vi "Virtual_Blink.vi"() -> ()   [LabVIEW 2020]
uses:
  <vilib>/Instr/_visa.llb/VISA Configure Serial Port (Instr).vi
panel:
  out "x = y?":bool
  out "read buffer 2":string
  out "read buffer":string
  in  "Start":bool
  in  "Stop":bool
  in  "Serial port configuration":T1
  in  "Port":refnum<visa-resource-name>
  out "Output LED":bool
  # "Project name:  Virtual_Blink.vi \nDescription:     Blink LED emulation using Intel Galileo board\nVersion:           02.00\nRevision:          00\nLast modified : 12/31/2020"
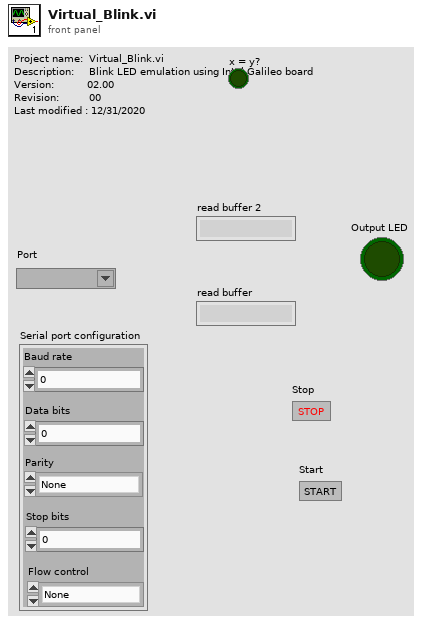
[diagram p1: front panel]
types:
  T1 = cluster{"Baud rate":u32, "Data bits":u16, "Parity":enum16{"None", "Odd", "Even", "Mark", "Space"}, "Stop bits":u16, "Flow control":enum32{"None", "XON/XOFF", "RTS/CTS", "DTR/DSR"}}
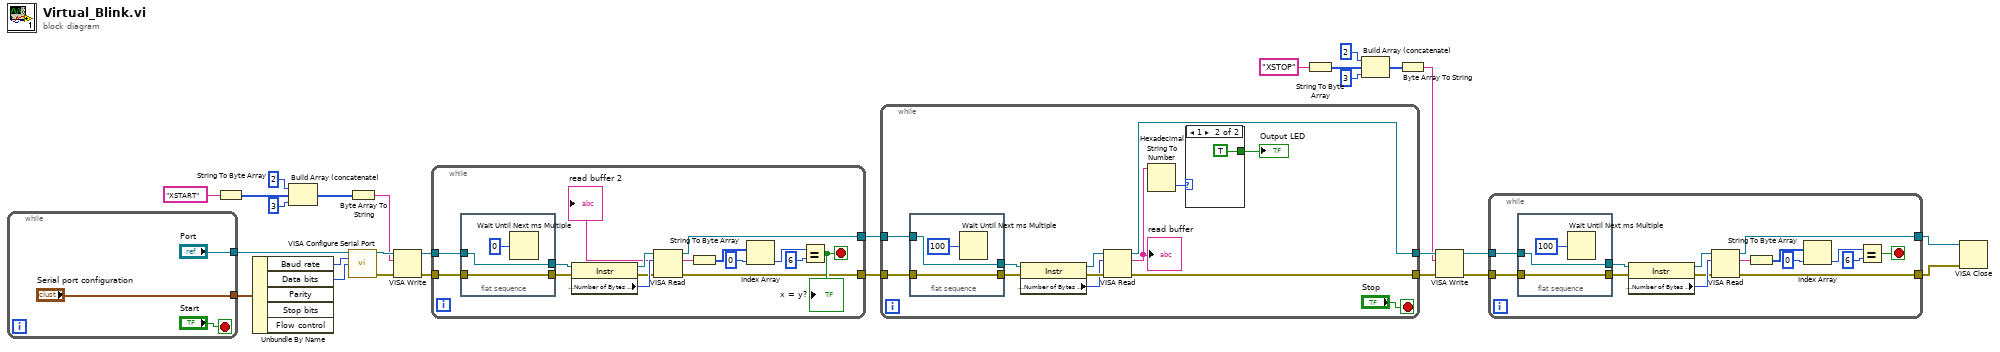
[diagram p0: block diagram]
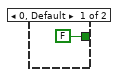
[diagram p2: hidden frame]
diagram:
  n1 = while {
    tunnel: ["Port"] -> w28
    tunnel: ["Serial port configuration"] -> w27
    stop <- "Start" stop-if-true
  }
  n2 = String To Byte Array(string="XSTART") -> (unsigned byte array=w20:u8[])
  n3 = Unbundle By Name(w27) -> ("Baud rate"=w26:u32, "Data bits"=w25:u16)  [unwired: 3 out]
  n4 = Build Array (concatenate)(u8 2, w20, u8 3) -> (w18:u8[])
  n5 = Byte Array To String(unsigned byte array=w18) -> (string=w17:string)
  n6 = call-poly "VISA Configure Serial Port"("VISA resource name"=w28, "baud rate (9600)"=w26, "data bits (8)"=w25) -> ("VISA resource name out"=w24:refnum<visa-resource-name>, "error out"=w23:errorcluster)  [unwired: 11 in]
  n7 = VISA Write(VISA resource name=w24, write buffer=w17, error in (no error)=w23) -> (VISA resource name out=w8:refnum<visa-resource-name>, error out=w7:errorcluster)  [unwired: 1 out]
  n8 = while {
    tunnel: w8 -> [w41]
    tunnel: w7 -> [w40]
    tunnel: [w33] -> w6
    tunnel: [w32] -> w5
    stop <- w34 stop-if-true
    n9 = flat-sequence {
      tunnel: w41 -> [w49]
      tunnel: w40 -> [w48]
      tunnel: [w49] -> w45
      tunnel: [w48] -> w46
      frame #0 {
        n10 = Wait Until Next ms Multiple(millisecond multiple=u32 0) -> ()  [unwired: 1 out]
      }
    }
    n11 = property class="Instr"(reference=w45, error in=w46) -> (reference out=w42:refnum<visa-resource-name>, error out=w43:errorcluster, "Serial Settings:Number of Bytes at Serial Port"=w44:u32)
    n12 = VISA Read(VISA resource name=w42, byte count=w44, error in (no error)=w43) -> (VISA resource name out=w33:refnum<visa-resource-name>, read buffer=w35:string, error out=w32:errorcluster)  [unwired: 1 out]
    "read buffer 2" <- w35
    n13 = String To Byte Array(string=w35) -> (unsigned byte array=w39:u8[])
    n14 = Index Array(array=w39, index=0) -> (element=w37:u8)
    n15 = Equal?(x=w37, y=u8 6) -> (x = y?=w34:bool)
    "x = y?" <- w34
  }
  n16 = while {
    tunnel: w6 -> [w53]
    tunnel: w5 -> [w52]
    tunnel: [w59] -> w10
    tunnel: [w58] -> w11
    stop <- "Stop" stop-if-true
    n17 = flat-sequence {
      tunnel: w53 -> [w64]
      tunnel: w52 -> [w63]
      tunnel: [w64] -> w51
      tunnel: [w63] -> w50
      frame #0 {
        n18 = Wait Until Next ms Multiple(millisecond multiple=u32 100) -> ()  [unwired: 1 out]
      }
    }
    n19 = property class="Instr"(reference=w51, error in=w50) -> (reference out=w56:refnum<visa-resource-name>, error out=w55:errorcluster, "Serial Settings:Number of Bytes at Serial Port"=w54:u32)
    n20 = VISA Read(VISA resource name=w56, byte count=w54, error in (no error)=w55) -> (VISA resource name out=w58:refnum<visa-resource-name>, read buffer=w57:string, error out=w59:errorcluster)  [unwired: 1 out]
    "read buffer" <- w57
    n21 = Hexadecimal String To Number(string=w57) -> (number=w62:u32)  [unwired: 2 in, 1 out]
    n22 = case shown="1" w62 {
      tunnel: [FALSE TRUE] -> w61
      frame 0, Default {
      }
      frame 1 {
      }
    }
    "Output LED" <- w61
  }
  n23 = String To Byte Array(string="XSTOP") -> (unsigned byte array=w14:u8[])
  n24 = Build Array (concatenate)(u8 2, w14, u8 3) -> (w12:u8[])
  n25 = Byte Array To String(unsigned byte array=w12) -> (string=w9:string)
  n26 = VISA Write(VISA resource name=w11, write buffer=w9, error in (no error)=w10) -> (VISA resource name out=w4:refnum<visa-resource-name>, error out=w3:errorcluster)  [unwired: 1 out]
  n27 = while {
    tunnel: w4 -> [w77]
    tunnel: w3 -> [w76]
    tunnel: [w69] -> w2
    tunnel: [w68] -> w1
    stop <- w70 stop-if-true
    n28 = flat-sequence {
      tunnel: w77 -> [w85]
      tunnel: w76 -> [w84]
      tunnel: [w85] -> w81
      tunnel: [w84] -> w82
      frame #0 {
        n29 = Wait Until Next ms Multiple(millisecond multiple=u32 100) -> ()  [unwired: 1 out]
      }
    }
    n30 = property class="Instr"(reference=w81, error in=w82) -> (reference out=w78:refnum<visa-resource-name>, error out=w79:errorcluster, "Serial Settings:Number of Bytes at Serial Port"=w80:u32)
    n31 = VISA Read(VISA resource name=w78, byte count=w80, error in (no error)=w79) -> (VISA resource name out=w69:refnum<visa-resource-name>, read buffer=w71:string, error out=w68:errorcluster)  [unwired: 1 out]
    n32 = String To Byte Array(string=w71) -> (unsigned byte array=w75:u8[])
    n33 = Index Array(array=w75, index=0) -> (element=w73:u8)
    n34 = Equal?(x=w73, y=u8 6) -> (x = y?=w70:bool)
  }
  n35 = VISA Close(VISA resource name=w2, error in (no error)=w1) -> ()  [unwired: 1 out]
